vi "CALCULA_Indices.vi"(10 "Start_end":i32[](array[numeric])=[2, 4, 7, 9], 11 "lineas_comando":i32=12) -> (1 "End 3":i32[](array[numeric])=[0, 1, 4, 3, 9, 5, 6, 0, 8, 0, 10, 11], 2 "Start 3":i32[](array[numeric])=[0, 1, 2, 3, 7, 5, 6, 0, 8, 0, 10, 11])   [LabVIEW 2017]
panel:
  out "Array 2":i32[](array[numeric])=[-1, -1, 0, -1, 1, -1, -1, 2, -1, 3, -1, -1]
  out "idx":i32=8
  out "idx_t":i32
  out "idx":i32
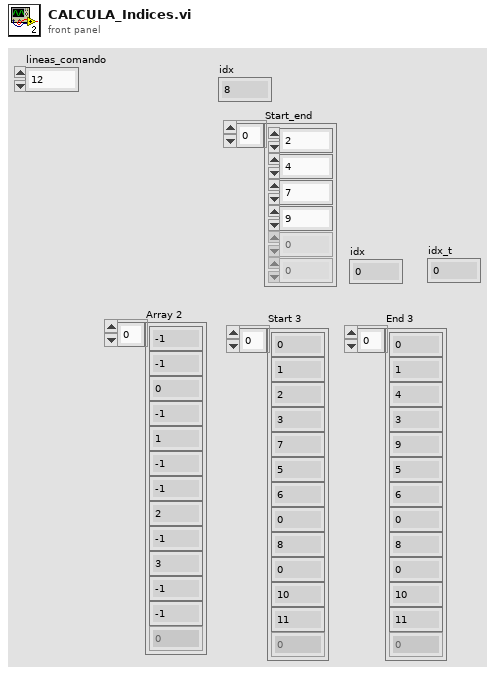
[diagram p1: front panel]
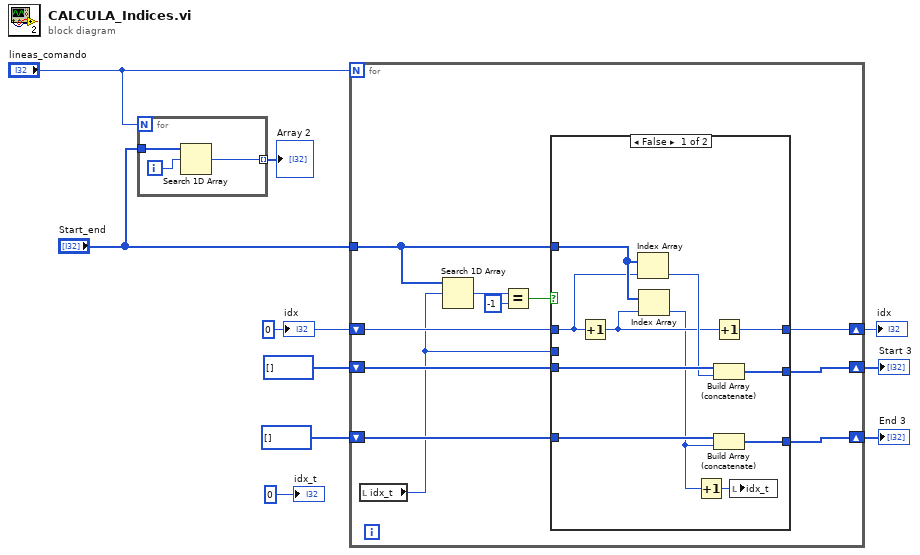
[diagram p0: block diagram]
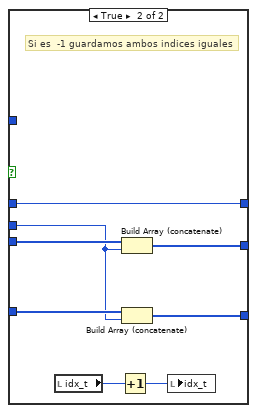
[diagram p2: hidden frame]
diagram:
  w8 = 0 ("idx")
  n1 = for {
    N: "lineas_comando" -> [_]
    tunnel: "Start_end" -> [w12]
    tunnel: [w11] -> w1 mode=indexing
    i -> [w13]
    n2 = Search 1D Array(1D array=w12, element=w13) -> (index of element=w11:i32)  [unwired: 1 in]
  }
  "Array 2" <- w1
  n3 = for {
    N: "lineas_comando" -> [_]
    tunnel: "Start_end" -> [w16]
    shift-right: [w21] -> w7
    shift-left: i32[] [] -> [w23]
    shift-right: [w20] -> w6
    shift-left: i32[] [] -> [w22]
    shift-right: [w19] -> w4
    shift-left: w8 -> [w15]
    n4 = local read "idx_t"() -> (w14:i32)
    n5 = Search 1D Array(1D array=w16, element=w14) -> (index of element=w17:i32)  [unwired: 1 in]
    n6 = Equal?(x=w17, y=-1) -> (x = y?=w24:bool)
    n7 = case shown="False" w24 {
      tunnel: w23 -> [w34 w43]
      tunnel: w22 -> [w35 w42]
      tunnel: [w32 w41] -> w20
      tunnel: [w33 w40] -> w21
      tunnel: w14 -> [_ w39]
      tunnel: [w31 w38] -> w19
      tunnel: w16 -> [w29 _]
      tunnel: w15 -> [w28 w38]
      frame False {
        n8 = Increment(x=w28) -> (x+1=w27:i32)
        n9 = Index Array(array=w29, index=w28) -> (element=w30:i32)
        n10 = Index Array(array=w29, index=w27) -> (element=w25:i32)
        n11 = Increment(x=w25) -> (x+1=w26:i32)
        n12 = Increment(x=w27) -> (x+1=w31:i32)
        n13 = Build Array (concatenate)(w34, w30) -> (w33:i32[])
        n14 = Build Array (concatenate)(w35, w25) -> (w32:i32[])
        n15 = local write "idx_t"(w26) -> ()
      }
      frame True {
        # "Si es  -1 guardamos ambos indices iguales"
        n16 = local read "idx_t"() -> (w37:i32)
        n17 = Increment(x=w37) -> (x+1=w36:i32)
        n18 = Build Array (concatenate)(w43, w39) -> (w40:i32[])
        n19 = Build Array (concatenate)(w42, w39) -> (w41:i32[])
        n20 = local write "idx_t"(w36) -> ()
      }
    }
  }
  "Start 3" <- w7
  "End 3" <- w6
  "idx" <- w4
  "idx" <- w8
  "idx_t" <- 0 ("idx tot")
